vi "Vacuum Tester 2.vi"() -> ()   [LabVIEW 2011]
panel:
  in  "stop":bool
  in  "Array":bool[](array[boolean])
  in  "lines":tag
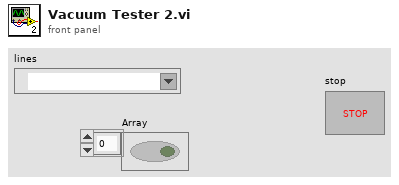
[diagram p1: front panel]
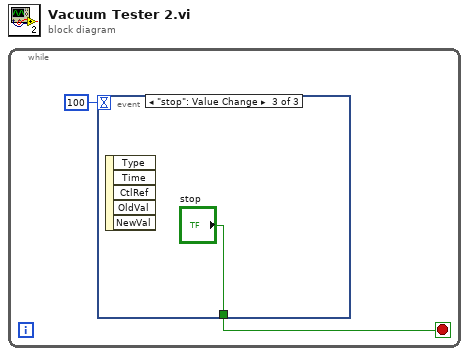
[diagram p0: block diagram]
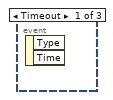
[diagram p2: hidden frame]
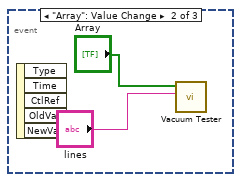
[diagram p3: hidden frame]
diagram:
  n1 = while {
    stop <- w1 stop-if-true
    n2 = event shown="[2] \"stop\": Value Change" {
      selector: _ -> [_ _ _]
      dyn-events: _ -> [_ _ _]
      timeout: 100 -> [_ _ _]
      tunnel: [_ _ "stop"] -> w1
      event Timeout {
        n3 = event-data() -> ()  [unwired: 1 in, 2 out]
      }
      event "Array": Value Change {
        n4 = event-data() -> ()  [unwired: 1 in, 5 out]
        n5 = call "Vacuum Tester.vi"("lines"="lines", "Pressure Controls"="Array") -> ()  [unwired: 8 in, 2 out]
      }
      event "stop": Value Change {
        n6 = event-data() -> ()  [unwired: 1 in, 5 out]
      }
    }
  }
